vi "Ophir SendReceive.vi"(3 "error in (no error)":errorcluster, 4 "Command":string, 5 "Visa Session":refnum<visa-resource-name>) -> (0 "error out":errorcluster, 1 "Frame Output":string, 2 "dup Visa Session":refnum<visa-resource-name>)   [LabVIEW 2017]
doc: "SendReceive.vi sends command to Instrument and returns the instrument's response.\nVersion 2.00 \nLast Updated 15 May 2002\n\nInputs:\nVisa Session\nCommand : String\nCommands examples : \"SP\" (Send Power) \"VE\" (VErsion) ..\ndefault empty string\nErrorIn\n\nOutputs:\ndup Visa Session\nFrame Output : String , Device Response to the Input Command\nErrorOut"
panel:
  out "return count":u32
  out "output string":string
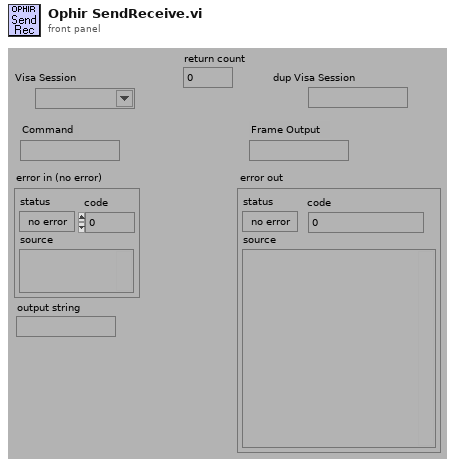
[diagram p1: front panel]
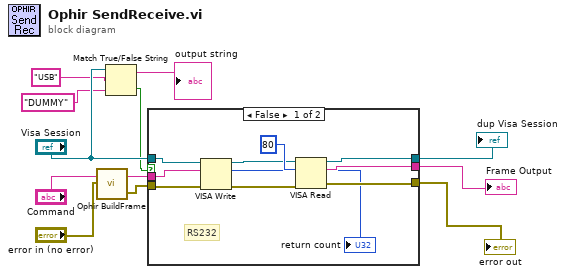
[diagram p0: block diagram]
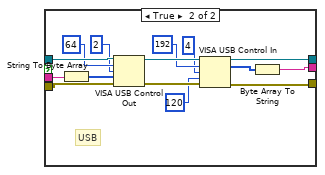
[diagram p2: hidden frame]
diagram:
  n1 = call "Ophir BuildFrame.vi"("error in (no error)"="error in (no error)", "Command Input"="Command") -> ("error out"=w7:errorcluster, "Output Frame"=w6:string)
  n2 = Match True/False String(2:"DUMMY", 3:"USB", 4:"Visa Session") -> (0:w3:bool, 1:→"output string":string)
  n3 = case shown="False" w3 {
    tunnel: "Visa Session" -> [w22 w35]
    tunnel: [w17 w26] -> w12
    tunnel: [w16 w25] -> w11
    tunnel: [w18 w23] -> w10
    tunnel: w7 -> [w21 w36]
    tunnel: w6 -> [w15 w37]
    frame False {
      # "RS232"
      n4 = VISA Write(VISA resource name=w22, write buffer=w15, error in (no error)=w21) -> (VISA resource name out=w19:refnum<visa-resource-name>, return count=→"return count":u32, error out=w14:errorcluster)
      n5 = VISA Read(VISA resource name=w19, byte count=u32 80, error in (no error)=w14) -> (VISA resource name out=w17:refnum<visa-resource-name>, read buffer=w18:string, error out=w16:errorcluster)  [unwired: 1 out]
    }
    frame True {
      # "USB"
      n6 = String To Byte Array(string=w37) -> (unsigned byte array=w32:u8[])
      n7 = VISA USB Control Out(0:w35, 5:i16 64 ("request type"), 7:i16 2 ("request"), 9:w32, 11:w36) -> (4:w31:refnum<visa-resource-name>, 15:w30:errorcluster)  [unwired: 2 out]
      n8 = VISA USB Control In(0:w31, 5:i16 192 ("request type"), 7:i16 4 ("request"), 9:u16 120 ("length (0)"), 11:w30) -> (4:w26:refnum<visa-resource-name>, 6:w24:u8[], 15:w25:errorcluster)  [unwired: 2 out]
      n9 = Byte Array To String(unsigned byte array=w24) -> (string=w23:string)
    }
  }
  "error out" <- w11
  "dup Visa Session" <- w12
  "Frame Output" <- w10
